vi "7.1-Make angle Array.vi"() -> (0 "Array":sgl[](array[numeric]))   [LabVIEW 2010]
uses:
  7.0-Global.vi
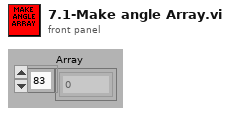
[diagram p1: front panel]
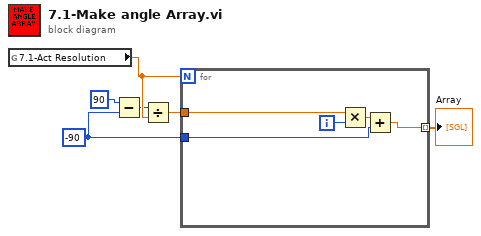
[diagram p0: block diagram]
diagram:
  w1 = -90 ("y")
  n1 = global read "7.0-Global.vi" "7.1-Act Resolution"() -> (w6:sgl)
  n2 = Subtract(x=90 ("y"), y=w1) -> (x-y=w3:i32)
  n3 = Divide(x=w3, y=w6) -> (x/y=w2:sgl)
  n4 = for {
    N: w6 -> [_]
    tunnel: w2 -> [w10]
    tunnel: w1 -> [w9]
    tunnel: [w7] -> w5 mode=indexing
    i -> [w8]
    n5 = Multiply(x=w10, y=w8) -> (x*y=w11:sgl)
    n6 = Add(x=w11, y=w9) -> (x+y=w7:sgl)
  }
  "Array" <- w5
